vi "Goal Adder GUI.vi"(8 "error in (no error)":errorcluster, 9 "Month":T1, 10 "YYYY":i32, 11 "Database.lvclass":refnum<class "Database.lvclass">) -> (0 "error out":errorcluster, 3 "Database.lvclass":refnum<class "Database.lvclass">)   [LabVIEW 2018]
uses:
  support/classes/database/Database.lvclass
  support/classes/database/Month.ctl
  support/classes/Category/Category.lvclass
panel:
  in  "Add":bool
  in  "Done":bool
  in  "Goal Amount":dbl
  in  "Category Table":i32(listbox)
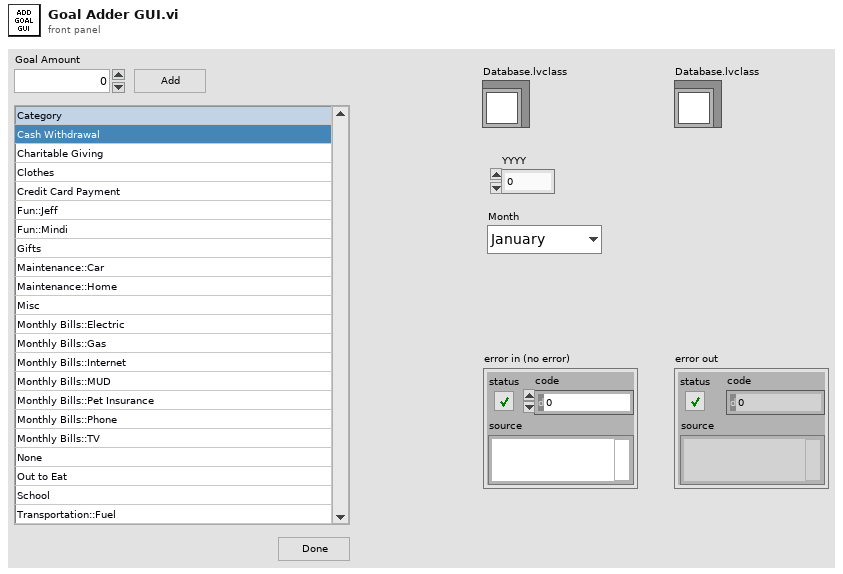
[diagram p1: front panel]
types:
  T1 = typedef "Database.lvclass/Month.ctl" = enum16{"January", "February", "March", "April", "May", "June", "July", "August", "September", "October", "November", "December"}
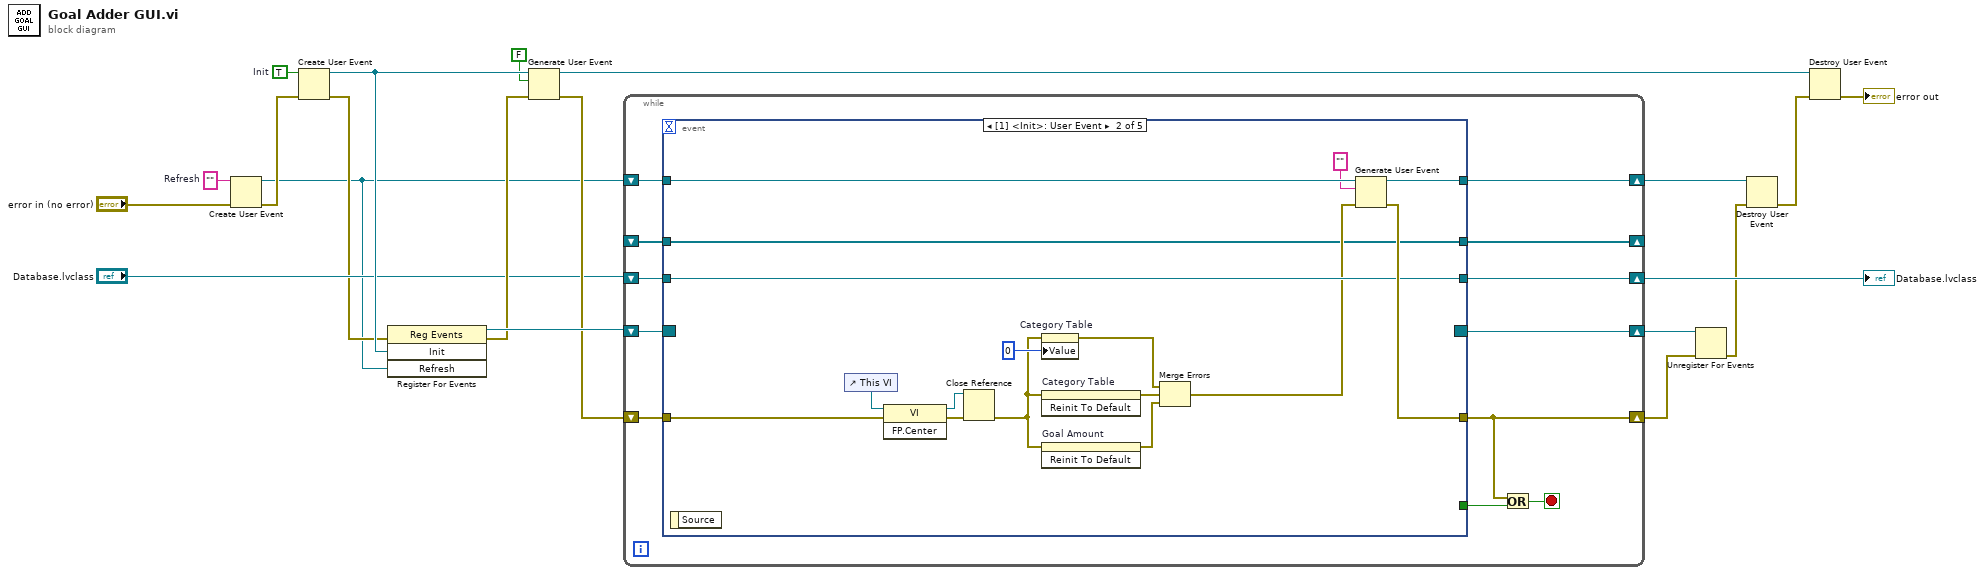
[diagram p0: block diagram]
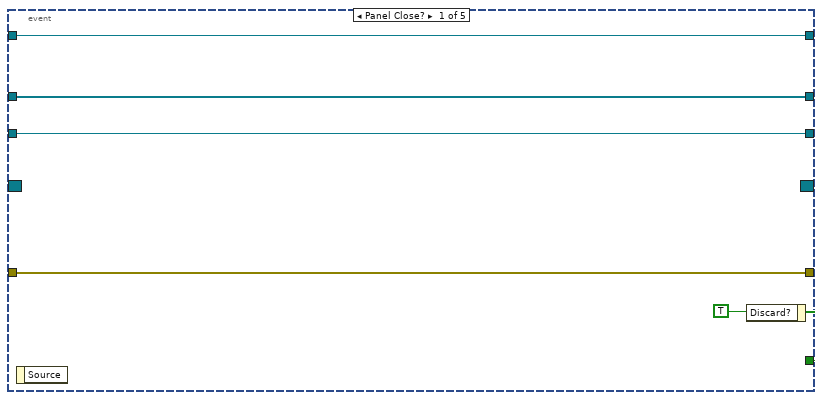
[diagram p2: hidden frame]
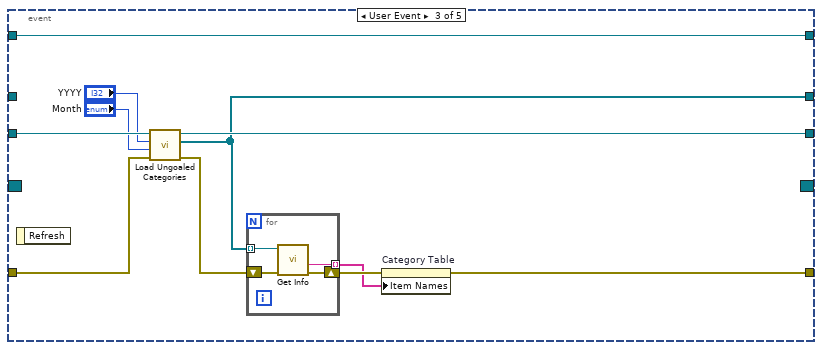
[diagram p3: hidden frame]
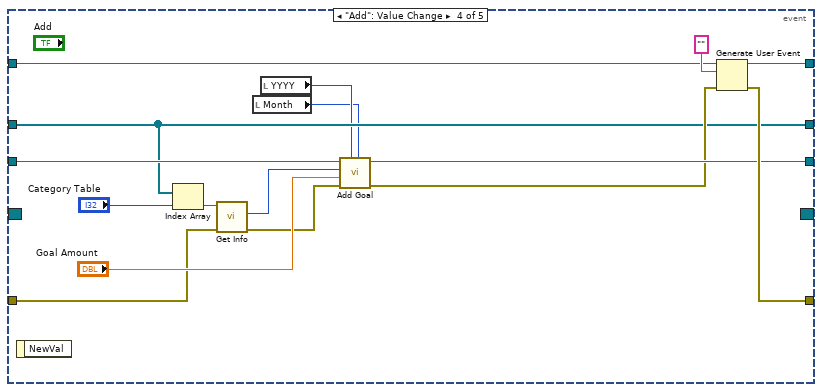
[diagram p4: hidden frame]
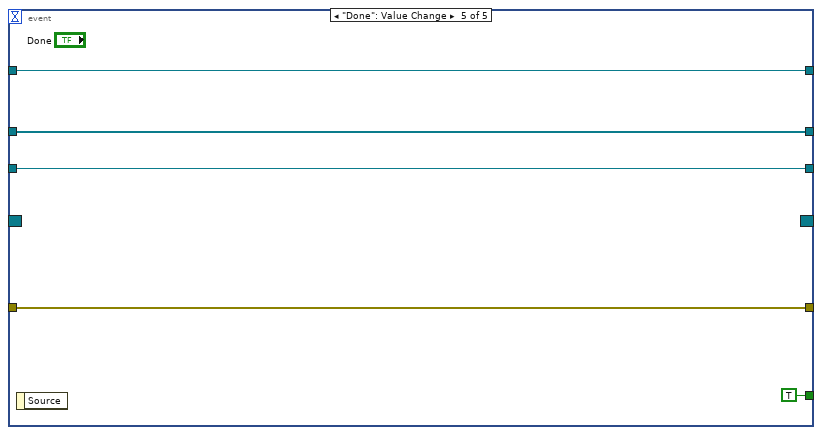
[diagram p5: hidden frame]
diagram:
  w1 = ""  # Refresh
  w20 = TRUE  # Init
  n1 = Create User Event(user event datatype=w1, error in="error in (no error)") -> (user event=w2:refnum<user-event>, error out=w4:errorcluster)
  n2 = Create User Event(user event datatype=w20, error in=w4) -> (user event=w18:refnum<user-event>, error out=w12:errorcluster)
  n3 = register-events(error in=w12, w18, w2) -> (reference out=w19:refnum<event-registration>, error out=w17:errorcluster)  [unwired: 1 in]
  n4 = Generate User Event(user event=w18, event data cluster=FALSE ("event data"), error in=w17) -> (user event out=w11:refnum<user-event>, error out=w16:errorcluster)  [unwired: 1 in]
  n5 = while {
    shift-right: [w30] -> w9
    shift-left: w19 -> [w32]
    shift-right: [w29] -> w8
    shift-left: w16 -> [w31]
    shift-right: [w25] -> w13
    shift-left: "Database.lvclass" -> [w26]
    shift-right: [w23] -> w5
    shift-left: w2 -> [w24]
    shift-right: [w22] -> _
    shift-left: _ -> [w21]
    stop <- w27 stop-if-true
    n6 = event shown="[1] <Init>: User Event" {
      selector: w32 -> [_ _ _ _ _]
      dyn-events: [_ _ _ _ _] -> w30
      timeout: _ -> [_ _ _ _ _]
      tunnel: [w37 _ _ _ TRUE ("Discard?")] -> w28
      tunnel: w31 -> [w36 w49 w60 w69 w86]
      tunnel: [w36 w42 w62 w81 w86] -> w29
      tunnel: w26 -> [w35 w40 w61 w80 w87]
      tunnel: [w35 w40 w58 w79 w87] -> w25
      tunnel: w24 -> [w34 w44 w64 w82 w88]
      tunnel: [w34 w43 w64 w83 w88] -> w23
      tunnel: [w33 w38 w54 w76 w85] -> w22
      tunnel: w21 -> [w33 w38 _ w76 w85]
      event Panel Close? {
        w37 = TRUE ("Discard?")
        n7 = event-data() -> ()  [unwired: 1 in, 1 out]
        n8 = event-data("Discard?"=w37) -> ()  [unwired: 1 in, 1 out]
      }
      event User Event {
        n9 = event-data() -> ()  [unwired: 1 in, 1 out]
        n10 = control-ref of="This VI"() -> (w50:refnum<vi>)
        n11 = invoke class="VI" method="FP.Center"(reference=w50, error in=w49) -> (reference out=w47:refnum<vi>, error out=w48:errorcluster)  [unwired: 1 in, 1 out]
        n12 = Close Reference(reference=w47, error in (no error)=w48) -> (error out=w46:errorcluster)
        n13 = property on="Category Table" class="LstBox (strict)"(error in=w46, "Value"=0 ("Category Table")) -> (error out=w45:errorcluster)  [unwired: 1 in, 1 out]
        n14 = invoke on="Category Table" class="LstBox (strict)" method="Reinit To Default"(error in=w46) -> (error out=w52:errorcluster)  [unwired: 2 in, 2 out]
        n15 = invoke on="Goal Amount" class="DigNum (strict)" method="Reinit To Default"(error in=w46) -> (error out=w53:errorcluster)  [unwired: 2 in, 2 out]
        n16 = Merge Errors(w45, w52, w53) -> (w39:errorcluster)
        n17 = Generate User Event(user event=w44, event data cluster="" ("event data"), error in=w39) -> (user event out=w43:refnum<user-event>, error out=w42:errorcluster)  [unwired: 1 in]
      }
      event User Event {
        n18 = event-data() -> ()  [unwired: 1 in, 1 out]
        n19 = call "Load Ungoaled Categories.vi"("error in (no error)"=w60, "Month"="Month", "YYYY"="YYYY", "Database in"=w61) -> ("error out"=w59:errorcluster, "Categories with No Goal"=w54:refnum<class "Category.lvclass">[], "Database out"=w58:refnum<class "Database.lvclass">)  [unwired: 5 in]
        n20 = for {
          shift-right: [w68] -> w63
          shift-left: w59 -> [w67]
          tunnel: w54 -> [w66] mode=indexing
          tunnel: [w65] -> w57 mode=indexing
          n21 = call "Get Info.vi"("error in (no error)"=w67, "Category in"=w66) -> ("error out"=w68:errorcluster, "Name"=w65:string)  [unwired: 6 in, 2 out]
        }
        n22 = property on="Category Table" class="LstBox (strict)"(error in=w63, "Item Names"=w57) -> (error out=w62:errorcluster)  [unwired: 1 in, 1 out]
      }
      event "Add": Value Change {
        n23 = event-data() -> ()  [unwired: 1 in, 1 out]
        n24 = Index Array(array=w76, index="Category Table") -> (element=w72:refnum<class "Category.lvclass">)
        n25 = call "Get Info.vi"("error in (no error)"=w69, "Category in"=w72) -> ("error out"=w70:errorcluster, "id"=w71:i32)  [unwired: 6 in, 2 out]
        n26 = local read "Month"() -> (w73:T1)
        n27 = local read "YYYY"() -> (w74:i32)
        n28 = call "Add Goal.vi"("Month"=w73, "YYYY"=w74, "error in (no error)"=w70, "Goal Amount"="Goal Amount", "Category_id"=w71, "Database in"=w80) -> ("error out"=w78:errorcluster, "Database out"=w79:refnum<class "Database.lvclass">)  [unwired: 4 in]
        n29 = Generate User Event(user event=w82, event data cluster="" ("event data"), error in=w78) -> (user event out=w83:refnum<user-event>, error out=w81:errorcluster)  [unwired: 1 in]
      }
      event "Done": Value Change {
        n30 = event-data() -> ()  [unwired: 1 in, 1 out]
      }
    }
    n31 = Or(x=w29, y=w28) -> (x .or. y?=w27:bool)
  }
  "Database.lvclass" <- w13
  n32 = Unregister For Events(event registration refnum=w9, error in=w8) -> (error out=w10:errorcluster)
  n33 = Destroy User Event(user event=w5, error in=w10) -> (error out=w7:errorcluster)
  n34 = Destroy User Event(user event=w11, error in=w7) -> (error out=→"error out":errorcluster)
